vi "Omron TCP FINS-Handshaking.vi"(8 "error in":errorcluster, 10 "Client IP":string, 11 "Buffer Data In":T1) -> (0 "error out":errorcluster, 3 "Buffer Data Out":T1)   [LabVIEW 2016]
uses:
  Data Def/Omron TCP FINS-Buffer Data.ctl
  Data Def/Omron TCP FINS-Command Code.ctl
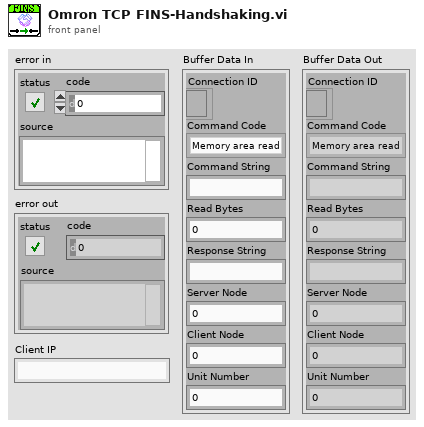
[diagram p1: front panel]
types:
  T1 = typedef "Omron TCP FINS-Buffer Data.ctl" = cluster{"Connection ID":refnum<k5>, "Command Code":T2, "Command String":string, "Read Bytes":i32, "Response String":string, "Server Node":u8, "Client Node":u8, "Unit Number":u8}
  T2 = typedef "Omron TCP FINS-Command Code.ctl" = enum16{"Memory area read", "Memory area write"}
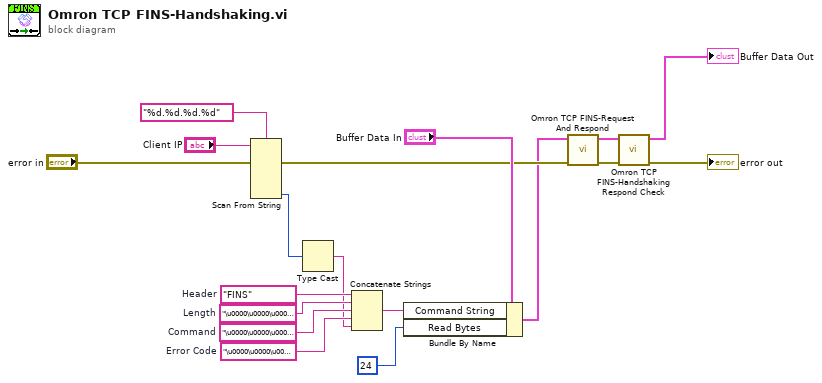
[diagram p0: block diagram]
diagram:
  w10 = "\u0000\u0000\u0000\u0000"  # Error Code
  w11 = "\u0000\u0000\u0000\u0000"  # Command
  w12 = "\u0000\u0000\u0000\f"  # Length
  w13 = "FINS"  # Header
  n1 = Scan From String(format string="%d.%d.%d.%d", input string="Client IP", error in="error in") -> (error out=w15:errorcluster, output 4=w14:i32)  [unwired: 8 in, 2 out]
  n2 = Type Cast(x=w14) -> (*(type *) &x=w9:string)  [unwired: 1 in]
  n3 = Concatenate Strings(w13, w12, w11, w10, w9) -> (w7:string)
  n4 = Bundle By Name(cluster="Buffer Data In", "Command String"=w7, "Read Bytes"=24) -> (w8:T1)
  n5 = call "Omron TCP FINS-Request And Respond.vi"("error in"=w15, "Buffer Data In"=w8) -> ("error out"=w5:errorcluster, "Buffer Data Out"=w2:T1)  [unwired: 8 in]
  n6 = call "Omron TCP FINS-Handshaking Respond Check.vi"("error in"=w5, "Buffer Data In"=w2) -> ("error out"=→"error out":errorcluster, "Buffer Data Out"=→"Buffer Data Out":T1)  [unwired: 8 in]
